vi "RUN.vi"() -> ()   [LabVIEW 2013]
uses:
  <userlib>/KNR OS 3.0 LabVIEW Toolkit/Type Definition/Resource.ctl
  <userlib>/KNR OS 3.0 LabVIEW Toolkit/Type Definition/DC Motor Port.ctl
  Global 1.vi
panel:
  in  "STOP 2":bool
  out "Battery\nVoltage":dbl format="%#_13g"
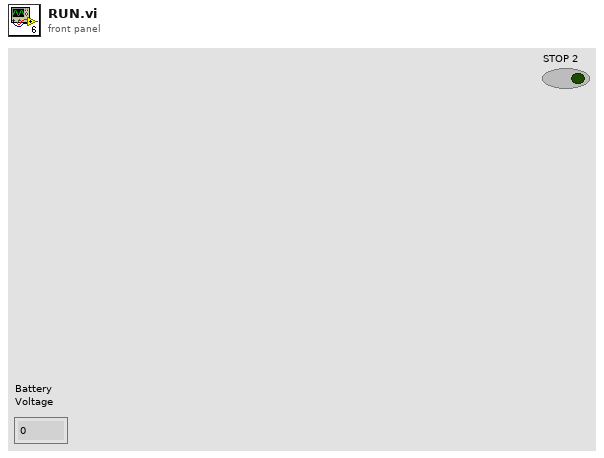
[diagram p1: front panel]
types:
  T1 = typedef "Resource.ctl" = enum16{"KNRm_DDRC", "KNRm_DDDD", "KNRm_DDDR", "KNRm_DDDC", "KNR"}
  T2 = typedef "KNR3 Reference.ctl" = cluster{"FPGA Session":refnum<class "FPGA Interface Base.lvclass">, "Resource":T1}
  T3 = typedef "DC Motor Port.ctl" = u16
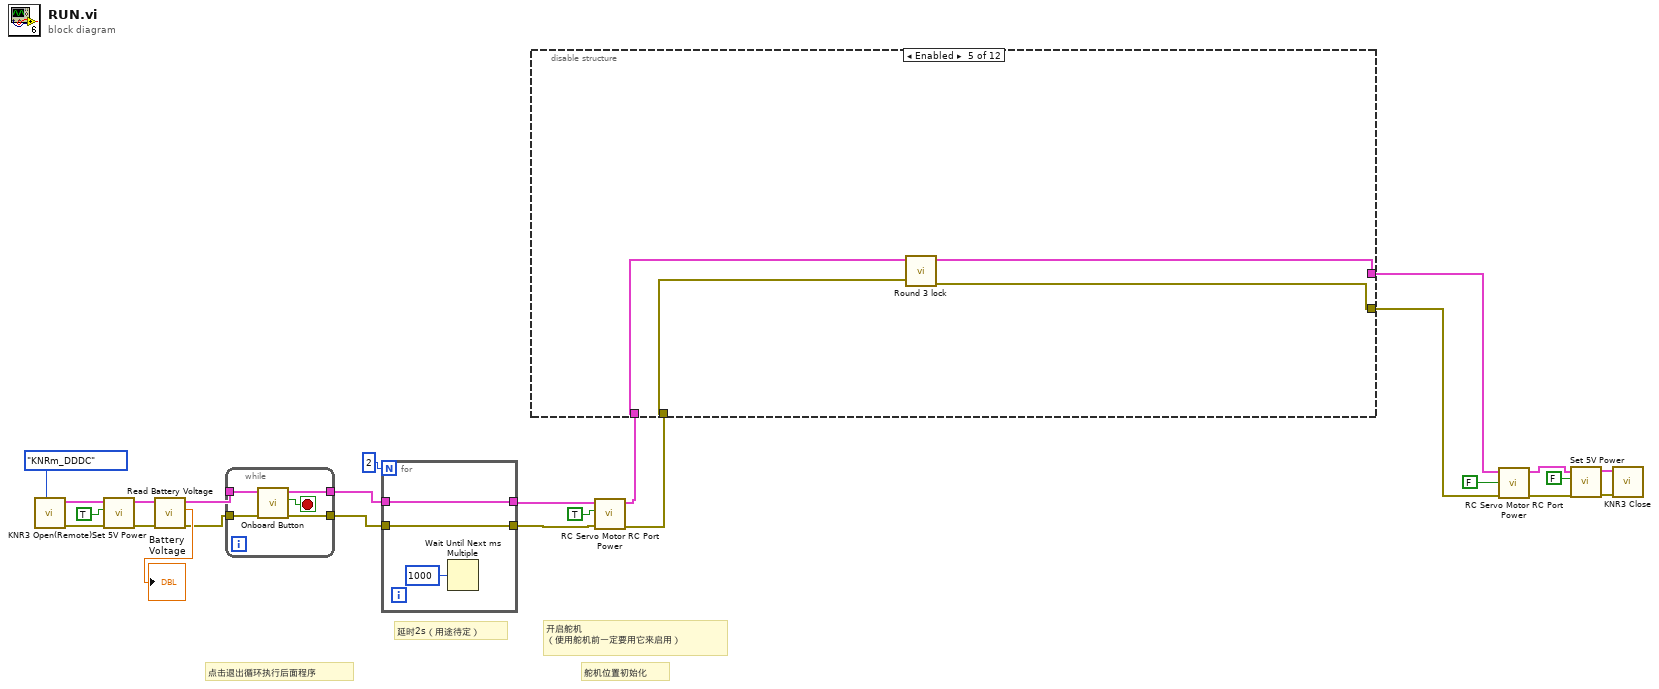
[diagram p0: block diagram]
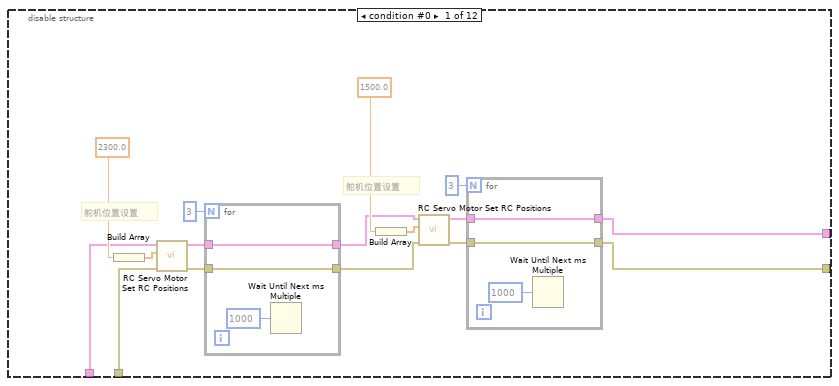
[diagram p2: hidden frame]
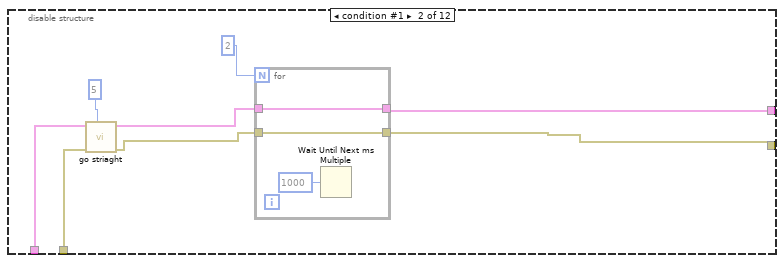
[diagram p3: hidden frame]
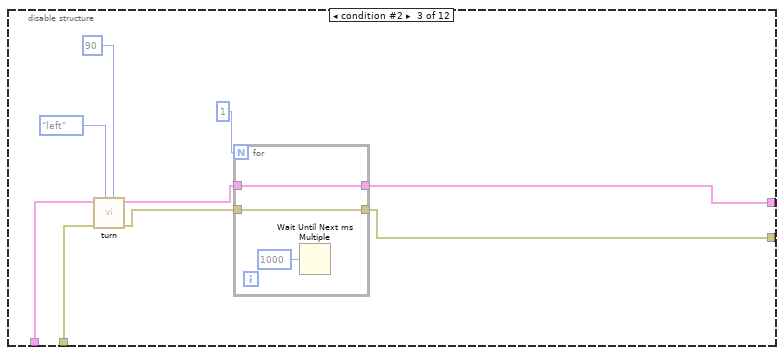
[diagram p4: hidden frame]
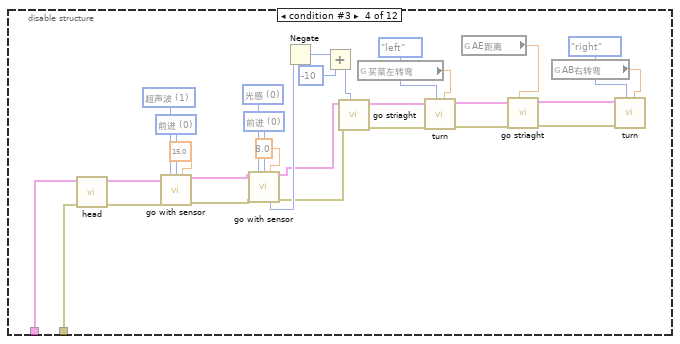
[diagram p5: hidden frame]
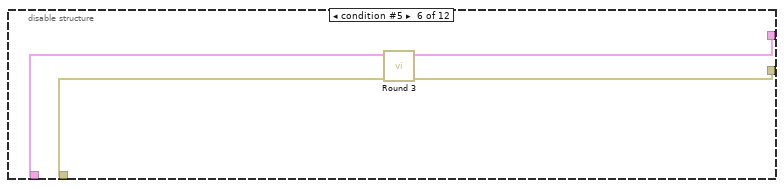
[diagram p6: hidden frame]
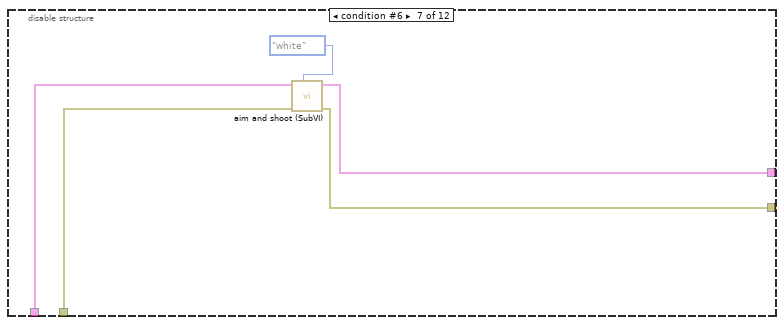
[diagram p7: hidden frame]
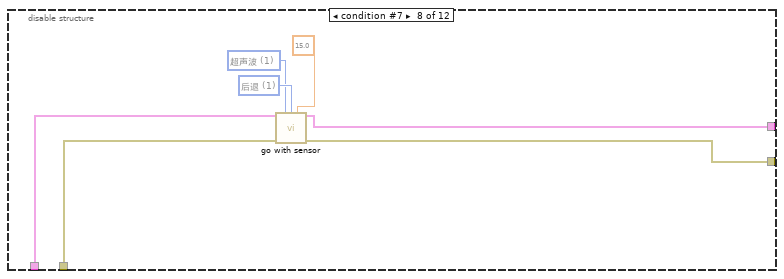
[diagram p8: hidden frame]
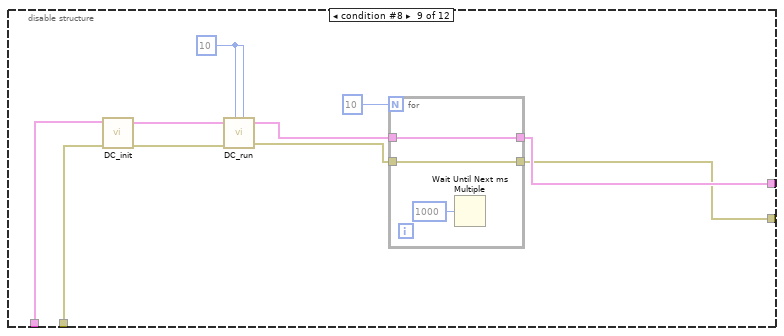
[diagram p9: hidden frame]
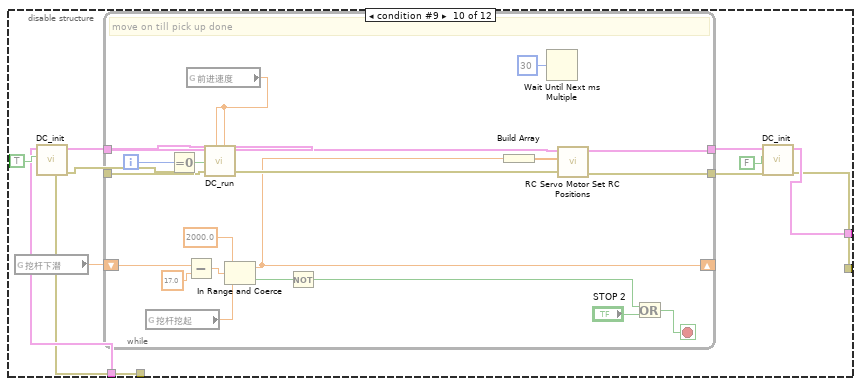
[diagram p10: hidden frame]
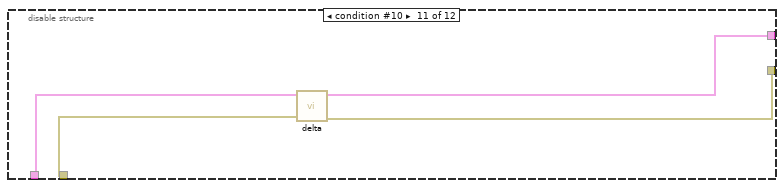
[diagram p11: hidden frame]
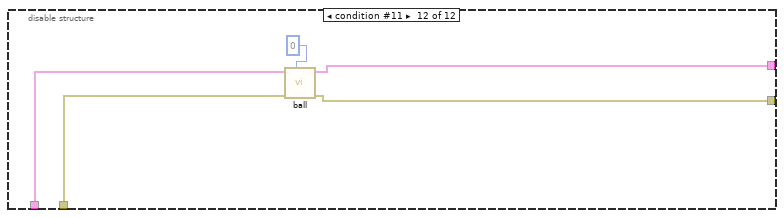
[diagram p12: hidden frame]
diagram:
  # "开启舵机\n（使用舵机前一定要用它来启用）"
  # "延时2s（用途待定）"
  # "舵机位置初始化"
  # "点击退出循环执行后面程序"
  n1 = call <userlib>:"KNR3 Open(Remote).vi"("Resource"=Resource."KNRm_DDDC") -> ("error out"=w23:errorcluster, "KNR out"=w24:T2)  [unwired: 9 in]
  n2 = call <userlib>:"Set 5V Power.vi"("error in (no error)"=w23, "5V Power(T)"=TRUE, "KNR in"=w24) -> ("error out"=w3:errorcluster, "KNR out"=w14:T2)  [unwired: 7 in]
  n3 = call <userlib>:"Read Battery Voltage.vi"("error in (no error)"=w3, "KNR in"=w14) -> ("error out"=w4:errorcluster, "Voltage"=→"Battery\nVoltage":dbl, "KNR out"=w5:T2)  [unwired: 7 in]
  n4 = while {
    tunnel: w5 -> [w30]
    tunnel: w4 -> [w29]
    tunnel: [w28] -> w2
    tunnel: [w27] -> w1
    stop <- w26 stop-if-true
    n5 = call <userlib>:"Onboard Button.vi"("error in (no error)"=w29, "KNR in"=w30) -> ("error out"=w27:errorcluster, "value"=w26:bool, "KNR out"=w28:T2)  [unwired: 7 in]
  }
  n6 = for {
    N: 2 -> [_]
    tunnel: w2 -> [w32]
    tunnel: w1 -> [w31]
    tunnel: [w31] -> w15
    tunnel: [w32] -> w16
    n7 = Wait Until Next ms Multiple(millisecond multiple=u32 1000) -> ()  [unwired: 1 out]
  }
  n8 = call <userlib>:"RC Servo Motor RC Port Power.vi"("error in (no error)"=w15, "RC Power(F)"=TRUE, "KNR in"=w16) -> ("error out"=w19:errorcluster, "KNR out"=w20:T2)  [unwired: 7 in]
  n9 = disable-structure shown="Enabled" {
    disable-tunnel: w20 -> [w47 w62 w74 w107 w111 w115 w118 w125 w137 w142 w176 w181]
    disable-tunnel: w19 -> [w46 w61 w73 w106 w110 w114 w117 w124 w136 w141 w175 w180]
    disable-tunnel: [w35 w57 w68 _ w109 w113 w120 w123 w130 w144 w174 w179] -> w7
    disable-tunnel: [w34 w56 w67 _ w108 w112 w119 w122 w129 w143 w173 w178] -> w6
    frame condition #0 {
      # "舵机位置设置"
      # "舵机位置设置"
      n10 = Build Array(2300.0 ("element")) -> (w48:dbl[])
      n11 = call <userlib>:"RC Servo Motor Set RC Positions.vi"("error in (no error)"=w46, "RC Pulse Width (1500 uS)"=w48, "KNR in"=w47) -> ("error out"=w44:errorcluster, "KNR out"=w45:T2)  [unwired: 7 in]
      n12 = for {
        N: 3 -> [_]
        tunnel: w45 -> [w54]
        tunnel: w44 -> [w55]
        tunnel: [w55] -> w36
        tunnel: [w54] -> w37
        n13 = Wait Until Next ms Multiple(millisecond multiple=u32 1000) -> ()  [unwired: 1 out]
      }
      n14 = Build Array(1500.0 ("element")) -> (w41:dbl[])
      n15 = call <userlib>:"RC Servo Motor Set RC Positions.vi"("error in (no error)"=w36, "RC Pulse Width (1500 uS)"=w41, "KNR in"=w37) -> ("error out"=w39:errorcluster, "KNR out"=w40:T2)  [unwired: 7 in]
      n16 = for {
        N: 3 -> [_]
        tunnel: w40 -> [w51]
        tunnel: w39 -> [w52]
        tunnel: [w52] -> w34
        tunnel: [w51] -> w35
        n17 = Wait Until Next ms Multiple(millisecond multiple=u32 1000) -> ()  [unwired: 1 out]
      }
    }
    frame condition #1 {
      n18 = call "go striaght.vi"("距离"=5, "error in (no error)"=w61, "KNR in"=w62) -> ("error out"=w58:errorcluster, "KNR out"=w59:T2)  [unwired: 7 in]
      n19 = for {
        N: 2 -> [_]
        tunnel: w59 -> [w65]
        tunnel: w58 -> [w66]
        tunnel: [w66] -> w56
        tunnel: [w65] -> w57
        n20 = Wait Until Next ms Multiple(millisecond multiple=u32 1000) -> ()  [unwired: 1 out]
      }
    }
    frame condition #2 {
      n21 = call "turn.vi"("Angle"=90, "side"=enum16{"right", "left"}."left", "error in (no error)"=w73, "KNR in"=w74) -> ("error out"=w69:errorcluster, "KNR out"=w70:T2)  [unwired: 6 in]
      n22 = for {
        N: 1 -> [_]
        tunnel: w70 -> [w77]
        tunnel: w69 -> [w78]
        tunnel: [w78] -> w67
        tunnel: [w77] -> w68
        n23 = Wait Until Next ms Multiple(millisecond multiple=u32 1000) -> ()  [unwired: 1 out]
      }
    }
    frame condition #3 {
      w99 = T3 0 items=["前进", "后退"] ("方向")
      w100 = T3 0 items=["光感", "超声波"] ("传感器类型")
      w104 = T3 0 items=["前进", "后退"] ("方向")
      w105 = T3 1 items=["光感", "超声波"] ("传感器类型")
      n24 = call "head.vi"("error in (no error)"=w106, "KNR in"=w107) -> ("error out"=w101:errorcluster, "KNR out"=w102:T2)  [unwired: 8 in]
      n25 = call "go with sensor.vi"("KNR in"=w102, "传感器类型"=w105, "方向"=w104, "then go:"=15.0, "error in (no error)"=w101) -> ("KNR out"=w97:T2, "error out"=w96:errorcluster)  [unwired: 8 in, 1 out]
      n26 = call "go with sensor.vi"("KNR in"=w97, "传感器类型"=w100, "方向"=w99, "then go:"=8.0, "error in (no error)"=w96) -> ("KNR out"=w81:T2, "offset"=w82:i32, "error out"=w80:errorcluster)  [unwired: 8 in]
      n27 = Negate(x=w82) -> (-x=w79:i32)
      n28 = Add(x=w79, y=-10) -> (x+y=w83:i32)
      n29 = call "go striaght.vi"("距离"=w83, "error in (no error)"=w80, "KNR in"=w81) -> ("error out"=w85:errorcluster, "KNR out"=w86:T2)  [unwired: 7 in]
      n30 = global read "Global 1.vi" "买菜左转弯"() -> (w94:dbl)
      n31 = call "turn.vi"("Angle"=w94, "side"=enum16{"right", "left"}."left", "error in (no error)"=w85, "KNR in"=w86) -> ("error out"=w87:errorcluster, "KNR out"=w88:T2)  [unwired: 6 in]
      n32 = global read "Global 1.vi" "AE距离"() -> (w91:dbl)
      n33 = call "go striaght.vi"("距离"=w91, "error in (no error)"=w87, "KNR in"=w88) -> ("error out"=w89:errorcluster, "KNR out"=w90:T2)  [unwired: 7 in]
      n34 = global read "Global 1.vi" "AB右转弯"() -> (w93:dbl)
      n35 = call "turn.vi"("Angle"=w93, "side"=enum16{"right", "left"}."right", "error in (no error)"=w89, "KNR in"=w90) -> ()  [unwired: 6 in, 2 out]
    }
    frame condition #4 (active) {
      n36 = call "Round 3 lock.vi"("error in (no error)"=w110, "KNR in"=w111) -> ("error out"=w108:errorcluster, "KNR out"=w109:T2)  [unwired: 8 in]
    }
    frame condition #5 {
      n37 = call "Round 3.vi"("error in (no error)"=w114, "KNR in"=w115) -> ("error out"=w112:errorcluster, "KNR out"=w113:T2)  [unwired: 8 in]
    }
    frame condition #6 {
      n38 = call "aim and shoot (SubVI).vi"("pin"=enum16{"white", "green", "left", "right"}."white", "error in (no error)"=w117, "KNR in"=w118) -> ("error out"=w119:errorcluster, "KNR out"=w120:T2)  [unwired: 7 in]
    }
    frame condition #7 {
      w127 = T3 1 items=["前进", "后退"] ("方向")
      w126 = T3 1 items=["光感", "超声波"] ("传感器类型")
      n39 = call "go with sensor.vi"("KNR in"=w125, "传感器类型"=w126, "方向"=w127, "then go:"=15.0, "error in (no error)"=w124) -> ("KNR out"=w123:T2, "error out"=w122:errorcluster)  [unwired: 8 in, 1 out]
    }
    frame condition #8 {
      w133 = 10
      n40 = call "DC_init.vi"("error in (no error)"=w136, "KNR in"=w137) -> ("error out"=w134:errorcluster, "KNR out"=w135:T2)  [unwired: 6 in, 2 out]
      n41 = call "DC_run.vi"("KNR in"=w135, "speed_1"=w133, "error in (no error)"=w134, "speed_2"=w133) -> ("KNR out"=w132:T2, "error out"=w131:errorcluster)  [unwired: 2 in, 2 out]
      n42 = for {
        N: 10 -> [_]
        tunnel: w132 -> [w139]
        tunnel: w131 -> [w140]
        tunnel: [w140] -> w129
        tunnel: [w139] -> w130
        n43 = Wait Until Next ms Multiple(millisecond multiple=u32 1000) -> ()  [unwired: 1 out]
      }
    }
    frame condition #9 {
      n44 = global read "Global 1.vi" "挖杆下潜"() -> (w145:dbl)
      n45 = call "DC_init.vi"("error in (no error)"=w141, "Enable Motor(T)"=TRUE, "KNR in"=w142) -> ("error out"=w146:errorcluster, "KNR out"=w147:T2)  [unwired: 5 in, 2 out]
      n46 = while {
        tunnel: w147 -> [w160]
        tunnel: w146 -> [w158]
        tunnel: [w163] -> w151
        tunnel: [w162] -> w150
        shift-right: [w154] -> _
        shift-left: w145 -> [w167]
        i -> [w170]
        stop <- w172 stop-if-true
        # "move on till pick up done"
        n47 = global read "Global 1.vi" "挖杆挖起"() -> (w155:dbl)
        n48 = Equal To 0?(x=w170) -> (x = 0?=w156:bool)
        n49 = Subtract(x=w167, y=17.0) -> (x-y=w165:dbl)
        n50 = global read "Global 1.vi" "前进速度"() -> (w161:dbl)
        n51 = call "DC_run.vi"("KNR in"=w160, "speed_1"=w161, "reinitialize? (F)"=w156, "error in (no error)"=w158, "speed_2"=w161) -> ("KNR out"=w159:T2, "error out"=w157:errorcluster)  [unwired: 1 in, 2 out]
        n52 = In Range and Coerce(upper limit=2000.0, x=w165, lower limit=w155) -> (coerced(x)=w154:dbl, In Range?=w153:bool)
        n53 = Not(x=w153) -> (.not. x?=w152:bool)
        n54 = Build Array(w154) -> (w168:dbl[])
        n55 = Wait Until Next ms Multiple(millisecond multiple=u32 30) -> ()  [unwired: 1 out]
        n56 = call <userlib>:"RC Servo Motor Set RC Positions.vi"("error in (no error)"=w157, "RC Pulse Width (1500 uS)"=w168, "KNR in"=w159) -> ("error out"=w162:errorcluster, "KNR out"=w163:T2)  [unwired: 7 in]
        n57 = Or(x=w152, y="STOP 2") -> (x .or. y?=w172:bool)
      }
      n58 = call "DC_init.vi"("error in (no error)"=w150, "Enable Motor(T)"=FALSE, "KNR in"=w151) -> ("error out"=w143:errorcluster, "KNR out"=w144:T2)  [unwired: 5 in, 2 out]
    }
    frame condition #10 {
      n59 = call "delta.vi"("error in (no error)"=w175, "KNR in"=w176) -> ("error out"=w173:errorcluster, "KNR out"=w174:T2)  [unwired: 8 in]
    }
    frame condition #11 {
      n60 = call "ball.vi"("Numeric"=0, "error in (no error)"=w180, "KNR in"=w181) -> ("error out"=w178:errorcluster, "KNR out"=w179:T2)  [unwired: 6 in, 1 out]
    }
  }
  n61 = call <userlib>:"RC Servo Motor RC Port Power.vi"("error in (no error)"=w6, "RC Power(F)"=FALSE, "KNR in"=w7) -> ("error out"=w8:errorcluster, "KNR out"=w9:T2)  [unwired: 7 in]
  n62 = call <userlib>:"Set 5V Power.vi"("error in (no error)"=w8, "5V Power(T)"=FALSE, "KNR in"=w9) -> ("error out"=w13:errorcluster, "KNR out"=w12:T2)  [unwired: 7 in]
  n63 = call <userlib>:"KNR3 Close.vi"("error in (no error)"=w13, "KNR in"=w12) -> ()  [unwired: 9 in, 1 out]
